vi "写盲元表到flash.vi"(8 "error in":errorcluster, 9 "data":u8[](array[numeric]), 10 "dwAddr":u32 format="%.0x", 11 "分辨率":string) -> (0 "error out":errorcluster, 2 "return":i32)   [LabVIEW 2016]
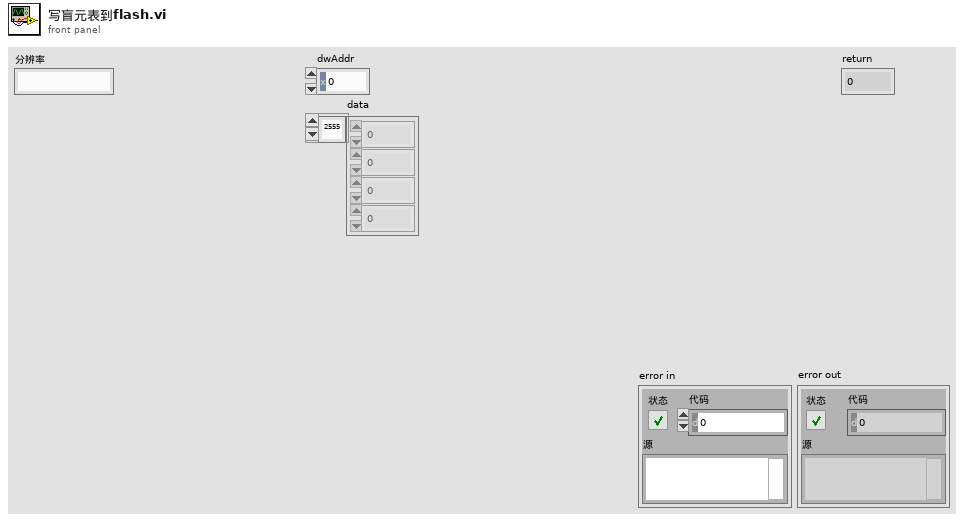
[diagram p1: front panel]
types:
  T1 = cluster{"byCmdType":u8, "bySubCmd":u8, "byPara":u8, "byAddr_h":u8, "byAddr_l":u8, "byAddr_ll":u8, "byLen_h":u8, "byLen_l":u8}
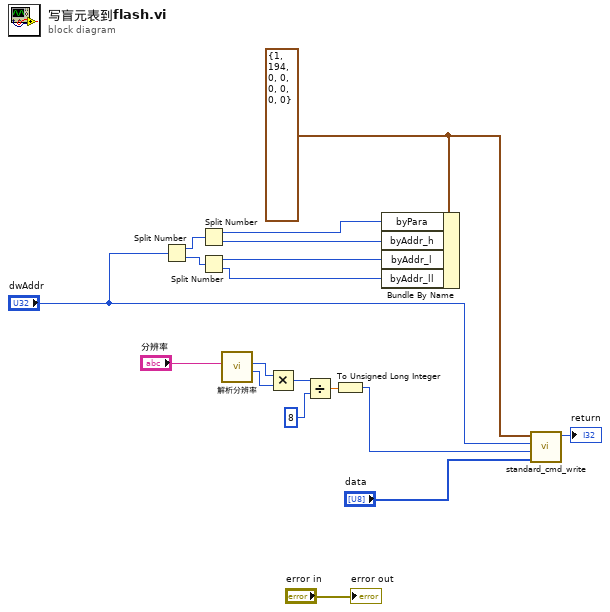
[diagram p0: block diagram]
diagram:
  w8 = T1 {"byCmdType"=1, "bySubCmd"=194, "byPara"=0, "byAddr_h"=0, "byAddr_l"=0, "byAddr_ll"=0, "byLen_h"=0, "byLen_l"=0} ("cmd_std_header_t")
  n1 = Split Number(x="dwAddr") -> (hi(x)=w6:u16, lo(x)=w5:u16)
  n2 = Split Number(x=w6) -> (hi(x)=w4:u8, lo(x)=w3:u8)
  n3 = Split Number(x=w5) -> (hi(x)=w2:u8, lo(x)=w1:u8)
  n4 = call "解析分辨率.vi"("分辨率"="分辨率") -> ("number 2"=w13:i32, "number"=w14:i32)  [unwired: 9 in]
  n5 = Multiply(x=w14, y=w13) -> (x*y=w12:i32)
  n6 = Divide(x=w12, y=8) -> (x/y=w10:dbl)
  n7 = To Unsigned Long Integer(number=w10) -> (unsigned 32bit integer=w9:u32)
  n8 = Bundle By Name(cluster=w8, "byPara"=w4, "byAddr_h"=w3, "byAddr_l"=w2, "byAddr_ll"=w1) -> ()  [unwired: 1 out]
  n9 = call "standard_cmd_write.vi"("data"="data", "dwLen"=w9, "dwAddr"="dwAddr", "cmd_std_header_t"=w8) -> ("return"=→"return":i32)  [unwired: 6 in, 1 out]
  "error out" <- "error in"
